vi "save configuration.vi"(8 "error in (no error)":errorcluster, 10 "Path":path, 11 "Camera":T1) -> (0 "error out":errorcluster, 3 "Camera out":T1)   [LabVIEW 2022 SP3, in "Vision.lvlib"]
uses:
  Vision.lvlib
  camera.ctl
  camera driver.ctl
  C:/Users/Caleb/Desktop/nebraska-silicon-lab/pixel-gantry-extra/LV/bin/uEyeDotNet.dll
  bin/uEyeDotNet.dll
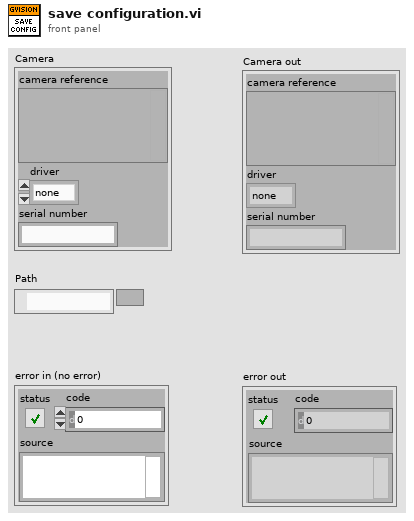
[diagram p1: front panel]
types:
  T1 = typedef "Vision.lvlib/camera.ctl" = cluster{"camera reference":variant, "driver":T2, "serial number":string}
  T2 = typedef "Vision.lvlib/camera driver.ctl" = enum16{"none", "ueye"}
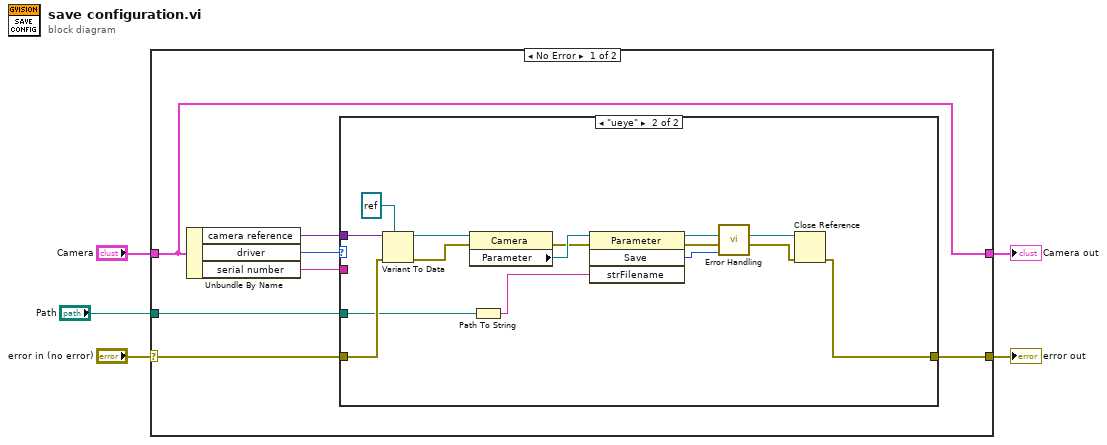
[diagram p0: block diagram]
diagram:
  n1 = case shown="No Error" "error in (no error)" {
    selector: "error in (no error)" -> [w7 w29]
    tunnel: [w9 w29] -> w4
    tunnel: "Camera" -> [w8 w28]
    tunnel: [w8 w28] -> w2
    tunnel: "Path" -> [w6 _]
    frame No Error {
      n2 = Unbundle By Name(w8) -> ("camera reference"=w11:variant, "driver"=w12:T2, "serial number"=w10:string)
      n3 = case shown="\"ueye\"" w12 {
        tunnel: w11 -> [_ w27]
        tunnel: w10 -> [_ _]
        tunnel: w7 -> [w13 w24]
        tunnel: [w13 w14] -> w9
        tunnel: w6 -> [_ w20]
        frame "none" {
        }
        frame "ueye" {
          n4 = Variant To Data(error in=w24, type=refnum<k24> refnum ("reference"), Variant=w27) -> (data=w25:refnum<k24>, error out=w23:errorcluster)
          n5 = property class="Camera"(reference=w25, error in=w23) -> (error out=w21:errorcluster, "Parameter"=w22:refnum<k24>)  [unwired: 1 out]
          n6 = Path To String(path=w20) -> (string=w19:string)
          n7 = invoke class="Parameter" method="Save"(reference=w22, error in=w21, "strFilename"=w19) -> (reference out=w16:refnum<k24>, error out=w17:errorcluster, "Save"=w18:i32)  [unwired: 1 in, 1 out]
          n8 = call "Error Handling.vi"("Error Code"=w18, "Error In"=w17) -> ("Error Out"=w15:errorcluster)  [unwired: 9 in]
          n9 = Close Reference(reference=w16, error in (no error)=w15) -> (error out=w14:errorcluster)
        }
      }
    }
    frame Error {
    }
  }
  "error out" <- w4
  "Camera out" <- w2
